vi "optionsFrame_PathsGlobal.vi"() -> ()   [LabVIEW 2016]
panel:
  in  "Page Paths":path[](array[path])
  in  "Page titles":string[](array[string])
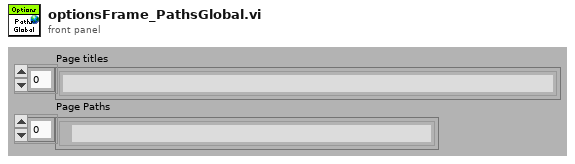
[diagram p1: front panel]
diagram:
